vi "myRIO_BRig_RT__Case_Exp_subState_LC__initTrial_subunit1_wrong.vi"(0 "input_LR_OnOff":bool, 2 "input_I_firstTrial":bool, 3 "input_spout":u16, 4 "input_randomNumber":u16, 5 "input_LR_Block":u16, 7 "input_LR_Trial":u16, 9 "input_LR_Probability":u16, 12 "input_iTrial":u16, 13 "input_nRewTrials":u16) -> (8 "output_LR_Event":bool, 10 "output_LR_Laser":bool)   [LabVIEW 2014]
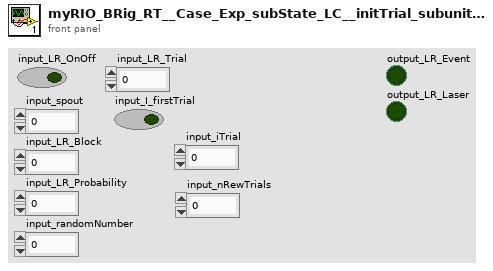
[diagram p1: front panel]
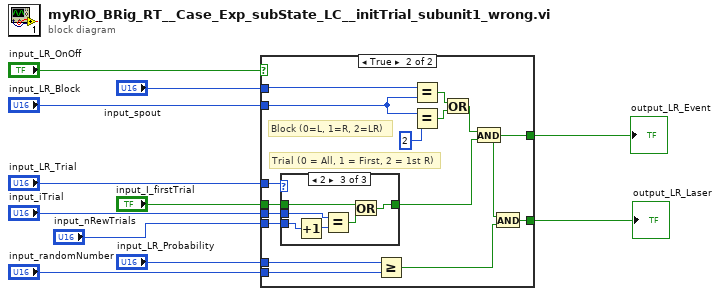
[diagram p0: block diagram]
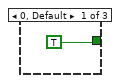
[diagram p3: hidden frame]
diagram:
  n1 = case shown="True" "input_LR_OnOff" {
    tunnel: "input_LR_Block" -> [_ w23]
    tunnel: "input_LR_Trial" -> [_ w16]
    tunnel: "input_LR_Probability" -> [_ w24]
    tunnel: [_ w20] -> w3
    tunnel: [_ w19] -> w4
    tunnel: "input_spout" -> [_ w18]
    tunnel: "input_I_firstTrial" -> [_ w15]
    tunnel: "input_randomNumber" -> [_ w17]
    tunnel: "input_iTrial" -> [_ w13]
    tunnel: "input_nRewTrials" -> [_ w12]
    frame False {
    }
    frame True {
      # "Block (0=L, 1=R, 2=LR)"
      # "Trial (0 = All, 1 = First, 2 = 1st R)"
      n2 = case shown="2" w16 {
        tunnel: [TRUE w29 w34] -> w14
        tunnel: w15 -> [_ w29 w35]
        tunnel: w13 -> [_ _ w31]
        tunnel: w12 -> [_ _ w33]
        frame 0, Default {
        }
        frame 1 {
        }
        frame 2 {
          n3 = Increment(x=w33) -> (x+1=w32:u16)
          n4 = Equal?(x=w31, y=w32) -> (x = y?=w30:bool)
          n5 = Or(x=w35, y=w30) -> (x .or. y?=w34:bool)
        }
      }
      n6 = Greater Or Equal?(x=w24, y=w17) -> (x >= y?=w22:bool)
      n7 = Equal?(x=w18, y=w23) -> (x = y?=w26:bool)
      n8 = Equal?(x=w23, y=u16 2) -> (x = y?=w25:bool)
      n9 = Or(x=w26, y=w25) -> (x .or. y?=w21:bool)
      n10 = And(x=w21, y=w14) -> (x .and. y?=w19:bool)
      n11 = And(x=w19, y=w22) -> (x .and. y?=w20:bool)
    }
  }
  "output_LR_Event" <- w4
  "output_LR_Laser" <- w3
